vi "Begin.vi"(8 "error in":errorcluster) -> (0 "error out":errorcluster)   [LabVIEW 2017]
doc: "Called before other user functions, this VI is expected to open initial I/O refnums, load in file data, and do all program initialization. Notice that the <B>error out</B> terminal is simply used for data flow. Wiring it to other structures or subVIs ensures that this VI runs first."
uses:
  <vilib>/Rock Robotics/WPI/DriverStation/WPI_DriverStationRobotMode2.ctl
  <vilib>/Rock Robotics/WPI/Joystick/WPI_JoystickDeviceEnum.ctl
  <vilib>/Rock Robotics/SystemInterfaces/DIO/FPGA_DIOPWMChannel.ctl
  <vilib>/Rock Robotics/SystemInterfaces/DIO/FPGA_DIOChannel.ctl
  <vilib>/Rock Robotics/WPI/Solenoid/WPI_SolenoidChannel.ctl
  <vilib>/Rock Robotics/SystemInterfaces/AI/FPGA_AIChannel.ctl
  <vilib>/Rock Robotics/SystemInterfaces/i2clib/i2c_bus.ctl
  Robot Global Data.vi
  <vilib>/Rock Robotics/WPI/MotorControl/WPI_MotorControlOpen VictorSP.vi
  <vilib>/Rock Robotics/WPI/Counter/WPI_CounterDigitalInputToDigitalSource.vi
  <vilib>/Rock Robotics/WPI/Solenoid/WPI_SolenoidOpenSingle.vi
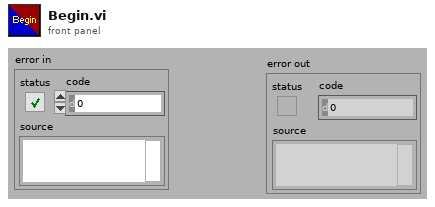
[diagram p1: front panel]
types:
  T1 = typedef "FPGA_DIOChannel.ctl" = enum8{"DIO 0", "DIO 1", "DIO 2", "DIO 3", "DIO 4", "DIO 5", "DIO 6", "DIO 7", "DIO 8", "DIO 9", "DIO MXP 0", "DIO MXP 1", "DIO MXP 2", "DIO MXP 3", "DIO MXP 4", "DIO MXP 5", "DIO MXP 6", "DIO MXP 7", "DIO MXP 8", "DIO MXP 9", "DIO MXP 10", "DIO MXP 11", "DIO MXP 12", "DIO MXP 13", "DIO MXP 14", "DIO MXP 15", "SPI Port CS1", "SPI Port CS2", "SPI Port CS3", "SPI Port MISO", "SPI Port MOSI", "Invalid"}
  T2 = typedef "WPI_JoystickDeviceEnum.ctl" = enum16{"USB 0", "USB 1", "USB 2", "USB 3", "USB 4", "USB 5"}
  T3 = typedef "i2c_bus.ctl" = enum16{"I2C On-Board", "I2C MXP", "Invalid"}
  T4 = typedef "FPGA_DIOPWMChannel.ctl" = enum8{"PWM 0", "PWM 1", "PWM 2", "PWM 3", "PWM 4", "PWM 5", "PWM 6", "PWM 7", "PWM 8", "PWM 9", "PWM MXP 0", "PWM MXP 1", "PWM MXP 2", "PWM MXP 3", "PWM MXP 4", "PWM MXP 5", "PWM MXP 6", "PWM MXP 7", "PWM MXP 8", "PWM MXP 9", "Invalid"}
  T5 = typedef "FPGA_AIChannel.ctl" = enum8{"AI 0", "AI 1", "AI 2", "AI 3", "AI MXP 0", "AI MXP 1", "AI MXP 2", "AI MXP 3", "Invalid"}
  T6 = typedef "WPI_SolenoidChannel.ctl" = enum8{"Solenoid 0", "Solenoid 1", "Solenoid 2", "Solenoid 3", "Solenoid 4", "Solenoid 5", "Solenoid 6", "Solenoid 7", "Invalid"}
  T7 = typedef "WPI_DriverStationRobotMode2.ctl" = enum16{"Autonomous Disabled", "Autonomous Enabled", "Teleop Disabled", "Teleop Enabled", "Disconnected", "Finish", "Test Disabled", "Test Enabled", "Emergency Stopped"}
  T8 = typedef "WPI_JoystickDevRef.ctl" = cluster{"Device":T2}
  T9 = typedef "WPI_DigitalInputDevRef.ctl" = cluster{"DevStatus":errorcluster, "DIO Channel":T1}
  T10 = typedef "WPI_I2CDevRef.ctl" = cluster{"DevStatus":errorcluster, "Device Address":u8, "Handle":i32, "I2C Bus":T3}
  T11 = typedef "FPGA_CounterEncoderSourceConvertionLVSourceType.ctl" = cluster{"DevStatus":errorcluster, "AnalogTriggerMode?":bool, "DigitalMode":cluster{"DIO Channel":T12}, "AnalogTriggerMode":cluster{"AnalogTriggerIndex":T13, "OutputType":T14}}
  T12 = typedef "FPGA_DIODigitalSourceChannel.ctl" = enum8{"DIO 0", "DIO 1", "DIO 2", "DIO 3", "DIO 4", "DIO 5", "DIO 6", "DIO 7", "DIO 8", "DIO 9", "DIO MXP 0", "DIO MXP 1", "DIO MXP 2", "DIO MXP 3", "DIO MXP 4", "DIO MXP 5", "DIO MXP 6", "DIO MXP 7", "DIO MXP 8", "DIO MXP 9", "DIO MXP 10", "DIO MXP 11", "DIO MXP 12", "DIO MXP 13", "DIO MXP 14", "DIO MXP 15", "Disabled"}
  T13 = typedef "FPGA_AnalogTriggerIndex.ctl" = enum8{"Trig 0", "Trig 1", "Trig 2", "Trig 3", "Trig 4", "Trig 5", "Trig 6", "Trig 7", "Invalid"}
  T14 = typedef "FPGA_AnalogTriggerOutType.ctl" = enum16{"InWindow", "TriggerState", "Rising", "Falling"}
  T15 = typedef "WPI_AnalogChannelDevRef.ctl" = cluster{"DevStatus":errorcluster, "Analog Channel":T5}
  T16 = typedef "WPI_EncoderDevRef.ctl" = cluster{"DevStatus":errorcluster, "EncoderIndex":T17, "CounterIndex":T18, "DistancePerCount":dbl, "Decoding Type":T19}
  T17 = typedef "FPGA_EncoderIdx.ctl" = enum8{"Enc 0", "Enc 1", "Enc 2", "Enc 3", "Enc 4", "Enc 5", "Enc 6", "Enc 7", "Invalid"}
  T18 = typedef "FPGA_CounterCtrSystemIndex.ctl" = enum8{"Ctr 0", "Ctr 1", "Ctr 2", "Ctr 3", "Ctr 4", "Ctr 5", "Ctr 6", "Ctr 7", "Invalid"}
  T19 = typedef "WPI_EncoderType.ctl" = enum16{"1x", "2x", "4x"}
  T20 = typedef "WPI_CompressorDevRef.ctl" = cluster{"DevStatus":errorcluster, "Pneumatics Control Module":u8}
  T21 = typedef "WPI_SolenoidDevRef.ctl" = cluster{"DevStatus":errorcluster, "Pneumatics Control Module":u8, "Forward Solenoid Channel":T6, "Reverse Solenoid Channel":T6}
  T22 = typedef "WPI_MotorControlDeviceRef.ctl" = cluster{"DeviceStatus":errorcluster, "Type":T23, "PWM":cluster{"PWM Channel":T4, "DeadBand":T24}, "CAN":cluster{"Device Number":u8, "SetOutput VI Ref":variant, "GetOutput VI Ref":variant, "Enable VI Ref":variant, "Disable VI Ref":variant, "Data":variant}, "Invert":bool, "DIO PWM":cluster{"PWM \"Enable\" Channel":T4, "DIOChannel":T1, "PWM Rate":dbl}}
  T23 = typedef "WPI_MotorControlType.ctl" = enum16{"PWM", "CAN", "DIO PWM"}
  T24 = typedef "WPI_PWMDeadband.ctl" = cluster{"Name":string, "maxPositivePwm":i32, "minPositivePwm":i32, "centerPwm":i32, "maxNegativePwm":i32, "minNegativePwm":i32, "angularRange":u16}
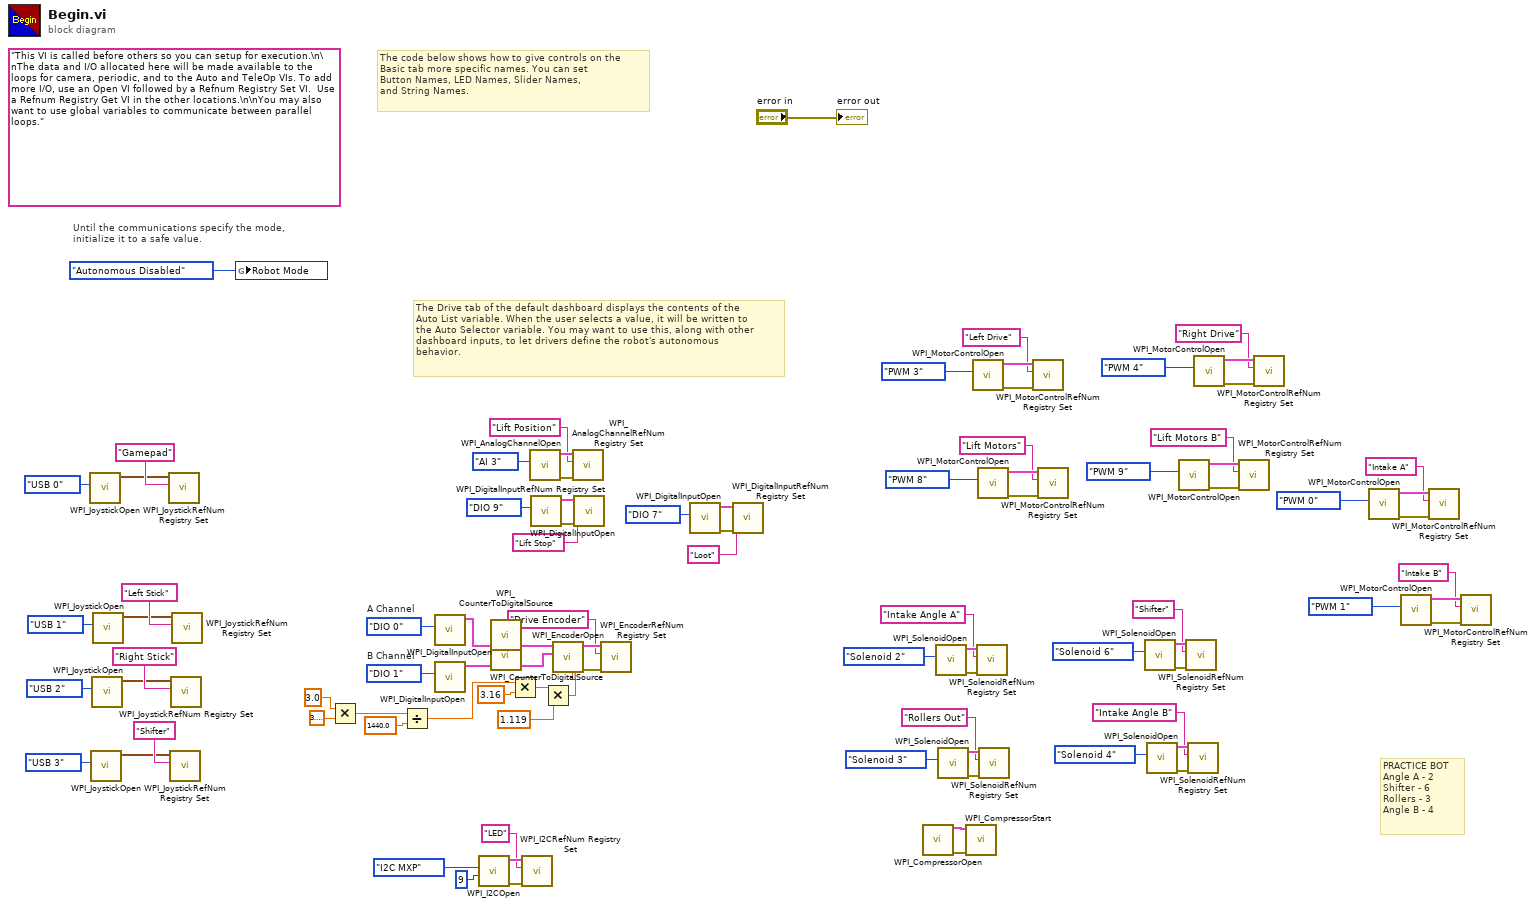
[diagram p0: block diagram]
diagram:
  w79 = FPGA_DIOChannel."DIO 1"  # B Channel
  w78 = FPGA_DIOChannel."DIO 0"  # A Channel
  (unwired) "This VI is called before others so you can setup for execution.\n\nThe data and I/O allocated here will be made available to the loops for camera, periodic, and to the Auto and TeleOp VIs. To add more I/O, use an Open VI followed by a Refnum Registry Set VI.  Use a Refnum Registry Get VI in the other locations.\n\nYou may also want to use global variables to communicate between parallel loops."
  # "PRACTICE BOT\nAngle A - 2\nShifter - 6\nRollers - 3\nAngle B - 4"
  # "The Drive tab of the default dashboard displays the contents of the\nAuto List variable. When the user selects a value, it will be written to\nthe Auto Selector variable. You may want to use this, along with other\ndashboard inputs, to let drivers define the robot's autonomous\nbehavior."
  # "The code below shows how to give controls on the\nBasic tab more specific names. You can set\nButton Names, LED Names, Slider Names,\nand String Names."
  # "Until the communications specify the mode,\ninitialize it to a safe value."
  n1 = call <vilib>:"WPI_JoystickOpen.vi"("JoystickDevice"=WPI_JoystickDeviceEnum."USB 0") -> ("JoystickDevRef"=w89:T8)  [unwired: 10 in]
  n2 = call <vilib>:"WPI_JoystickOpen.vi"("JoystickDevice"=WPI_JoystickDeviceEnum."USB 3") -> ("JoystickDevRef"=w6:T8)  [unwired: 10 in]
  n3 = call <vilib>:"WPI_JoystickOpen.vi"("JoystickDevice"=WPI_JoystickDeviceEnum."USB 2") -> ("JoystickDevRef"=w12:T8)  [unwired: 10 in]
  n4 = call <vilib>:"WPI_JoystickOpen.vi"("JoystickDevice"=WPI_JoystickDeviceEnum."USB 1") -> ("JoystickDevRef"=w9:T8)  [unwired: 10 in]
  n5 = call <vilib>:"WPI_JoystickRefNum Registry Set.vi"("refnum name"="Gamepad", "JoystickDevRef"=w89) -> ()  [unwired: 8 in, 2 out]
  n6 = call <vilib>:"WPI_JoystickRefNum Registry Set.vi"("refnum name"="Shifter", "JoystickDevRef"=w6) -> ()  [unwired: 8 in, 2 out]
  n7 = call <vilib>:"WPI_JoystickRefNum Registry Set.vi"("refnum name"="Right Stick", "JoystickDevRef"=w12) -> ()  [unwired: 8 in, 2 out]
  n8 = call <vilib>:"WPI_JoystickRefNum Registry Set.vi"("refnum name"="Left Stick", "JoystickDevRef"=w9) -> ()  [unwired: 8 in, 2 out]
  n9 = global write "Robot Global Data.vi" "Robot Mode"(WPI_DriverStationRobotMode2."Autonomous Disabled" ("Robot Mode")) -> ()
  n10 = Multiply(x=3.0, y=3.141592653589793) -> (x*y=w65:dbl)
  n11 = Divide(x=w65, y=1440.0) -> (x/y=w62:dbl)
  n12 = call <vilib>:"WPI_DigitalInputOpen.vi"("DIO Channel"=w78) -> ("DigitalInputDevRef"=w75:T9)  [unwired: 1 in, 9 out]
  n13 = call <vilib>:"WPI_DigitalInputOpen.vi"("DIO Channel"=w79) -> ("DigitalInputDevRef"=w76:T9)  [unwired: 1 in, 9 out]
  n14 = call <vilib>:"WPI_I2COpen.vi"("Device Address"=u8 9, "I2C Bus"=i2c_bus."I2C MXP") -> ("error out"=w22:errorcluster, "I2CDevRef"=w21:T10)  [unwired: 8 in]
  n15 = call-poly <vilib>:"WPI_CounterToDigitalSource.vi"("DigitalInputDevRef"=w75) -> ("Digital Source"=w74:T11)  [unwired: 6 out]
  n16 = call-poly <vilib>:"WPI_CounterToDigitalSource.vi"("DigitalInputDevRef"=w76) -> ("Digital Source"=w77:T11)  [unwired: 6 out]
  n17 = Multiply(x=w62, y=3.16) -> (x*y=w37:dbl)
  n18 = call <vilib>:"WPI_I2CRefNum Registry Set.vi"("error in (no error)"=w22, "refnum name"="LED", "I2CDevRef"=w21) -> ()  [unwired: 7 in, 2 out]
  n19 = call <vilib>:"WPI_AnalogChannelOpen.vi"("Analog Channel"=FPGA_AIChannel."AI 3") -> ("error out"=w33:errorcluster, "AIDeviceRef"=w32:T15)  [unwired: 9 in]
  n20 = call <vilib>:"WPI_DigitalInputOpen.vi"("DIO Channel"=FPGA_DIOChannel."DIO 9") -> ("error out"=w16:errorcluster, "DigitalInputDevRef"=w15:T9)  [unwired: 9 in]
  n21 = Multiply(x=w37, y=1.119) -> (x*y=w35:dbl)
  n22 = call <vilib>:"WPI_EncoderOpen.vi"("DistancePerCount"=w35, "BSource"=w77, "ASource"=w74) -> ("error out"=w73:errorcluster, "EncoderDevRef"=w72:T16)  [unwired: 5 in, 2 out]
  n23 = call <vilib>:"WPI_AnalogChannelRefNum Registry Set.vi"("error in (no error)"=w33, "refnum name"="Lift Position", "AIDeviceRef"=w32) -> ()  [unwired: 7 in, 2 out]
  n24 = call <vilib>:"WPI_DigitalInputRefNum Registry Set.vi"("error in (no error)"=w16, "refnum name"="Lift Stop", "DigitalInputDevRef"=w15) -> ()  [unwired: 7 in, 2 out]
  n25 = call <vilib>:"WPI_EncoderRefNum Registry Set.vi"("error in (no error)"=w73, "refnum name"="Drive Encoder", "EncoderDevRef"=w72) -> ()  [unwired: 7 in, 2 out]
  n26 = call <vilib>:"WPI_DigitalInputOpen.vi"("DIO Channel"=FPGA_DIOChannel."DIO 7") -> ("error out"=w3:errorcluster, "DigitalInputDevRef"=w1:T9)  [unwired: 9 in]
  n27 = call <vilib>:"WPI_DigitalInputRefNum Registry Set.vi"("error in (no error)"=w3, "refnum name"="Loot", "DigitalInputDevRef"=w1) -> ()  [unwired: 7 in, 2 out]
  n28 = call <vilib>:"WPI_CompressorOpen.vi"() -> ("CompressorDevRef"=w55:T20, "error out"=w54:errorcluster)  [unwired: 14 in]
  n29 = call-poly <vilib>:"WPI_SolenoidOpen.vi"("Solenoid Channel"=WPI_SolenoidChannel."Solenoid 2") -> ("error out"=w59:errorcluster, "SolenoidDevRef"=w58:T21)  [unwired: 9 in]
  n30 = call-poly <vilib>:"WPI_SolenoidOpen.vi"("Solenoid Channel"=WPI_SolenoidChannel."Solenoid 3") -> ("error out"=w49:errorcluster, "SolenoidDevRef"=w48:T21)  [unwired: 9 in]
  n31 = call <vilib>:"WPI_CompressorStart.vi"("error in (no error)"=w54, "CompressorDevRef"=w55) -> ()  [unwired: 8 in, 2 out]
  n32 = call-poly <vilib>:"WPI_MotorControlOpen.vi"("PWM Channel"=FPGA_DIOPWMChannel."PWM 3") -> ("error out"=w83:errorcluster, "MotorControlDeviceRef"=w82:T22)  [unwired: 9 in]
  n33 = call <vilib>:"WPI_SolenoidRefNum Registry Set.vi"("error in (no error)"=w59, "refnum name"="Intake Angle A", "SolenoidDevRef"=w58) -> ()  [unwired: 7 in, 2 out]
  n34 = call-poly <vilib>:"WPI_MotorControlOpen.vi"("PWM Channel"=FPGA_DIOPWMChannel."PWM 8") -> ("error out"=w70:errorcluster, "MotorControlDeviceRef"=w69:T22)  [unwired: 9 in]
  n35 = call <vilib>:"WPI_SolenoidRefNum Registry Set.vi"("error in (no error)"=w49, "refnum name"="Rollers Out", "SolenoidDevRef"=w48) -> ()  [unwired: 7 in, 2 out]
  n36 = call <vilib>:"WPI_MotorControlRefNum Registry Set.vi"("error in (no error)"=w83, "refnum name"="Left Drive", "MotorControlDevRef"=w82) -> ()  [unwired: 7 in, 2 out]
  n37 = call <vilib>:"WPI_MotorControlRefNum Registry Set.vi"("error in (no error)"=w70, "refnum name"="Lift Motors", "MotorControlDevRef"=w69) -> ()  [unwired: 7 in, 2 out]
  n38 = call-poly <vilib>:"WPI_SolenoidOpen.vi"("Solenoid Channel"=WPI_SolenoidChannel."Solenoid 6") -> ("error out"=w53:errorcluster, "SolenoidDevRef"=w52:T21)  [unwired: 9 in]
  n39 = call-poly <vilib>:"WPI_SolenoidOpen.vi"("Solenoid Channel"=WPI_SolenoidChannel."Solenoid 4") -> ("error out"=w45:errorcluster, "SolenoidDevRef"=w44:T21)  [unwired: 9 in]
  n40 = call-poly <vilib>:"WPI_MotorControlOpen.vi"("PWM Channel"=FPGA_DIOPWMChannel."PWM 9") -> ("error out"=w26:errorcluster, "MotorControlDeviceRef"=w25:T22)  [unwired: 9 in]
  n41 = call <vilib>:"WPI_SolenoidRefNum Registry Set.vi"("error in (no error)"=w53, "refnum name"="Shifter", "SolenoidDevRef"=w52) -> ()  [unwired: 7 in, 2 out]
  n42 = call <vilib>:"WPI_SolenoidRefNum Registry Set.vi"("error in (no error)"=w45, "refnum name"="Intake Angle B", "SolenoidDevRef"=w44) -> ()  [unwired: 7 in, 2 out]
  n43 = call-poly <vilib>:"WPI_MotorControlOpen.vi"("PWM Channel"=FPGA_DIOPWMChannel."PWM 4") -> ("error out"=w87:errorcluster, "MotorControlDeviceRef"=w86:T22)  [unwired: 9 in]
  n44 = call <vilib>:"WPI_MotorControlRefNum Registry Set.vi"("error in (no error)"=w26, "refnum name"="Lift Motors B", "MotorControlDevRef"=w25) -> ()  [unwired: 7 in, 2 out]
  n45 = call <vilib>:"WPI_MotorControlRefNum Registry Set.vi"("error in (no error)"=w87, "refnum name"="Right Drive", "MotorControlDevRef"=w86) -> ()  [unwired: 7 in, 2 out]
  n46 = call-poly <vilib>:"WPI_MotorControlOpen.vi"("PWM Channel"=FPGA_DIOPWMChannel."PWM 0") -> ("error out"=w41:errorcluster, "MotorControlDeviceRef"=w40:T22)  [unwired: 9 in]
  n47 = call-poly <vilib>:"WPI_MotorControlOpen.vi"("PWM Channel"=FPGA_DIOPWMChannel."PWM 1") -> ("error out"=w30:errorcluster, "MotorControlDeviceRef"=w29:T22)  [unwired: 9 in]
  n48 = call <vilib>:"WPI_MotorControlRefNum Registry Set.vi"("error in (no error)"=w41, "refnum name"="Intake A", "MotorControlDevRef"=w40) -> ()  [unwired: 7 in, 2 out]
  n49 = call <vilib>:"WPI_MotorControlRefNum Registry Set.vi"("error in (no error)"=w30, "refnum name"="Intake B", "MotorControlDevRef"=w29) -> ()  [unwired: 7 in, 2 out]
  "error out" <- "error in"
